vi "LaserLineDetection_Intensity_DrawLine.vi"(4 "Color":u32(colorbox)=16776960, 6 "Region of Interest (Rectangle)":T1, 8 "error in (no error)":errorcluster, 9 "intercept":dbl, 10 "slope":dbl, 11 "Refnum in":T2) -> (0 "error out":errorcluster, 3 "Image Out":T2)   [LabVIEW 2013]
uses:
  <vilib>/vision/Image Controls.llb/IMAQ Image.ctl
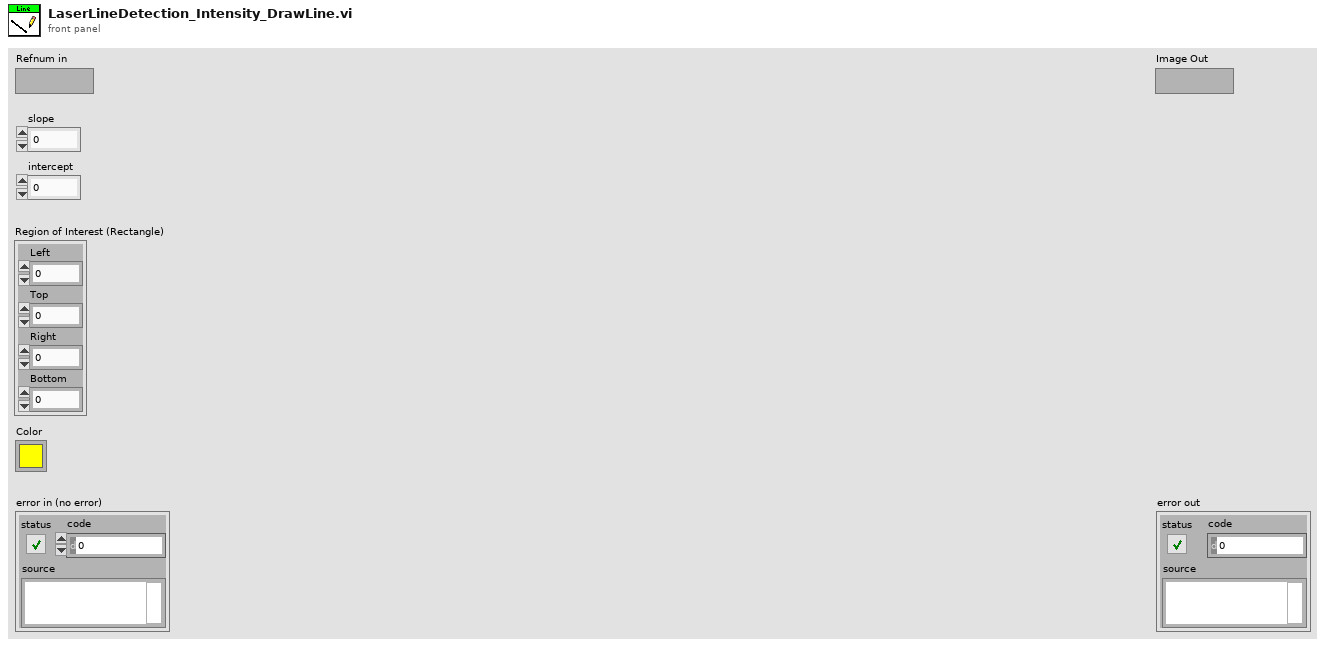
[diagram p1: front panel]
types:
  T1 = cluster{"Left":i32, "Top":i32, "Right":i32, "Bottom":i32}
  T2 = typedef "IMAQ Image.ctl" = refnum<image>
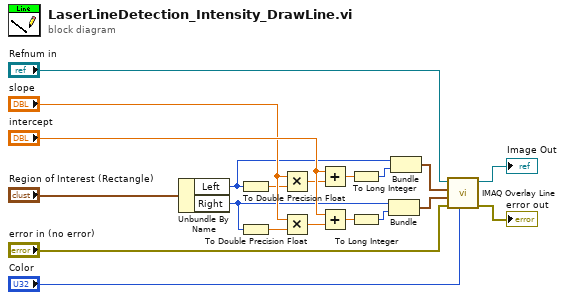
[diagram p0: block diagram]
diagram:
  n1 = Unbundle By Name("Region of Interest (Rectangle)") -> ("Left"=w13:i32, "Right"=w11:i32)
  n2 = To Double Precision Float(number=w13) -> (double precision float=w7:dbl)
  n3 = To Double Precision Float(number=w11) -> (double precision float=w5:dbl)
  n4 = Multiply(x="slope", y=w7) -> (x*y=w9:dbl)
  n5 = Multiply(x="slope", y=w5) -> (x*y=w3:dbl)
  n6 = Add(x="intercept", y=w9) -> (x+y=w8:dbl)
  n7 = Add(x="intercept", y=w3) -> (x+y=w4:dbl)
  n8 = To Long Integer(number=w8) -> (32bit integer=w10:i32)
  n9 = To Long Integer(number=w4) -> (32bit integer=w12:i32)
  n10 = Bundle("Right"=w11, w12) -> (w2:cluster{"Right":i32, i32})  [unwired: 1 in]
  n11 = Bundle("Left"=w13, w10) -> (w1:cluster{"Left":i32, i32})  [unwired: 1 in]
  n12 = call "IMAQ Overlay Line"("Color"="Color", "error in (no error)"="error in (no error)", "End Point"=w2, "Start Point"=w1, "Image"="Refnum in") -> ("error out"=→"error out":errorcluster, "Image Out"=→"Image Out":T2)  [unwired: 5 in]
